vi "Find Timer From Refnum.vi"(4 "Timers out":T1(array[cluster]) {"Total time (s)" format="%.2f"; "Start time (s)" format="%.2f"}, 5 "timer refnum":u32, 8 "timer name":string) -> (0 "timer refnum out":u32, 1 "Found":bool, 2 "timer index":i32, 3 "name out":string)   [LabVIEW 2011]
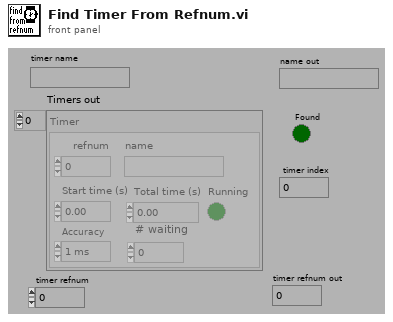
[diagram p1: front panel]
types:
  T1 = cluster{"refnum":u32, "Start time (s)":dbl, "Running":bool, "Total time (s)":dbl, "name":string, "Accuracy":enum16{"1 ms", "10 ms"}, "# waiting":i32}[]
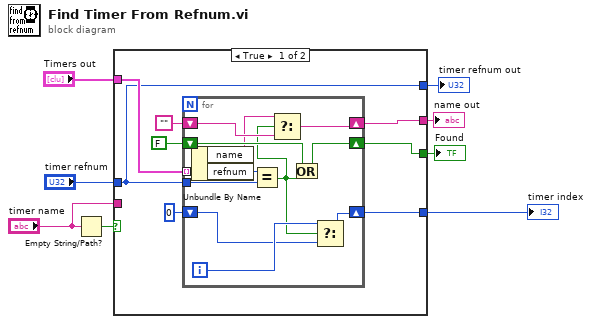
[diagram p0: block diagram]
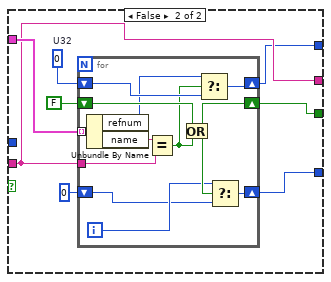
[diagram p2: hidden frame]
diagram:
  n1 = Empty String/Path?(string/path="timer name") -> (empty?=w3:bool)
  n2 = case shown="True" w3 {
    tunnel: [w16 w36] -> w8
    tunnel: "Timers out" -> [w15 w35]
    tunnel: [w13 w30] -> w6
    tunnel: [w11 w33] -> w5
    tunnel: "timer refnum" -> [w9 _]
    tunnel: "timer name" -> [_ w30]
    tunnel: [w9 w29] -> w1
    frame True {
      n3 = for {
        tunnel: w15 -> [w25] mode=indexing
        tunnel: w9 -> [w27]
        shift-right: [w18] -> w11
        shift-left: FALSE -> [w26]
        shift-right: [w22] -> w13
        shift-left: "" -> [w24]
        shift-right: [w19] -> w16
        shift-left: 0 -> [w20]
        i -> [w21]
        n4 = Unbundle By Name(w25) -> ("name"=w23:string, "refnum"=w28:u32)
        n5 = Equal?(x=w28, y=w27) -> (x = y?=w17:bool)
        n6 = Select(t=w23, s=w17, f=w24) -> (s? t:f=w22:string)
        n7 = Or(x=w26, y=w17) -> (x .or. y?=w18:bool)
        n8 = Select(t=w21, s=w17, f=w20) -> (s? t:f=w19:i32)
      }
    }
    frame False {
      w31 = u32 0  # U32
      n9 = for {
        tunnel: w35 -> [w44] mode=indexing
        tunnel: w30 -> [w47]
        shift-right: [w45] -> w33
        shift-left: FALSE -> [w46]
        shift-right: [w41] -> w29
        shift-left: w31 -> [w43]
        shift-right: [w37] -> w36
        shift-left: 0 -> [w38]
        i -> [w39]
        n10 = Unbundle By Name(w44) -> ("refnum"=w42:u32, "name"=w48:string)
        n11 = Equal?(x=w48, y=w47) -> (x = y?=w40:bool)
        n12 = Or(x=w46, y=w40) -> (x .or. y?=w45:bool)
        n13 = Select(t=w42, s=w40, f=w43) -> (s? t:f=w41:u32)
        n14 = Select(t=w39, s=w45, f=w38) -> (s? t:f=w37:i32)
      }
    }
  }
  "timer index" <- w8
  "name out" <- w6
  "Found" <- w5
  "timer refnum out" <- w1
